vi "ABF1_Read.vi"(4 "에러 입력":errorcluster, 7 "FilePath":path=path "C:/Users/KimYG/Experimental Data/Flocculus_Ex vivo/6. Plsticity/190119/190119_#07/190119__0026.abf") -> (0 "error out":errorcluster caption="에러 출력", 2 "Header":T1)   [LabVIEW 2017]
uses:
  ABF1FIO.lvclass
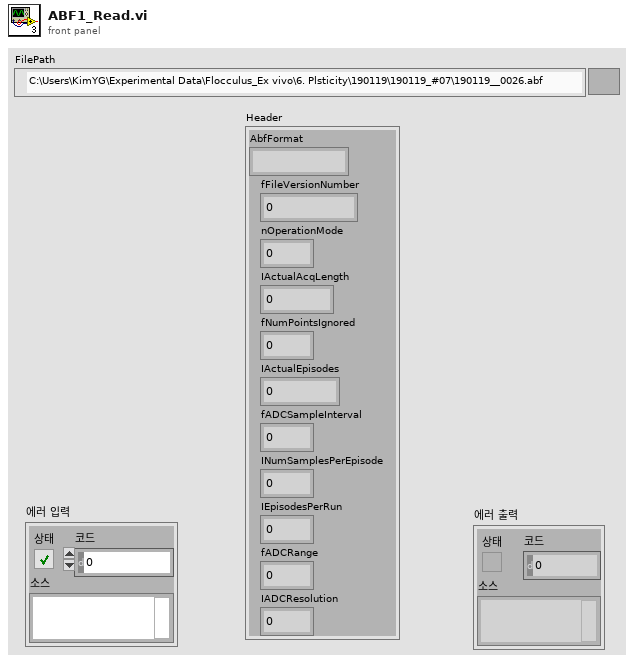
[diagram p1: front panel]
types:
  T1 = cluster{"AbfFormat":string, "fFileVersionNumber":sgl, "nOperationMode":i8, "IActualAcqLength":u32, "fNumPointsIgnored":i8, "IActualEpisodes":i32, "fADCSampleInterval":sgl, "INumSamplesPerEpisode":u32, "IEpisodesPerRun":u32, "fADCRange":sgl, "IADCResolution":u32}
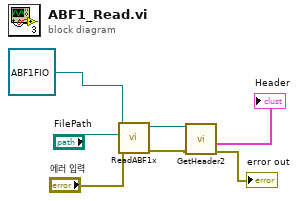
[diagram p0: block diagram]
diagram:
  n1 = call-dynamic "ReadABF1x.vi"("error in (no error)"="에러 입력", "FilePath"="FilePath", "ABF1FIO 입력"=refnum<class "ABF1FIO.lvclass"> refnum ("ABF1FIO.lvclass")) -> ("error out"=w3:errorcluster, "ABF1FIO 출력"=w4:refnum<class "ABF1FIO.lvclass">)  [unwired: 7 in]
  n2 = call-dynamic "GetHeader2.vi"("error in (no error)"=w3, "ABF1FIO 입력"=w4) -> ("error out"=→"error out":errorcluster, "Header"=→"Header":T1)  [unwired: 7 in, 1 out]
